vi "test.vi"() -> ()   [LabVIEW 2018]
uses:
  Content/TypeDef/EventTypeDef.ctl
  HASS-LV-WS_integration.lvlib
  <vilib>/MediaMongrels Ltd/WebSockets/WebSockets/WebSockets.lvlib
panel:
  out "States":T1(array[cluster])
  in  "Fetch states":bool
  out "Success":bool
  in  "Call Service Data":T2
  in  "call service btn":bool
  out "Event Data":string
  in  "Remove Button":bool
  in  "Add Button":bool
  in  "Event":string
  out "Event Name":string
  in  "Stop Button":bool
  out "Connection Authenticated?":bool
  out "Connection Result":string
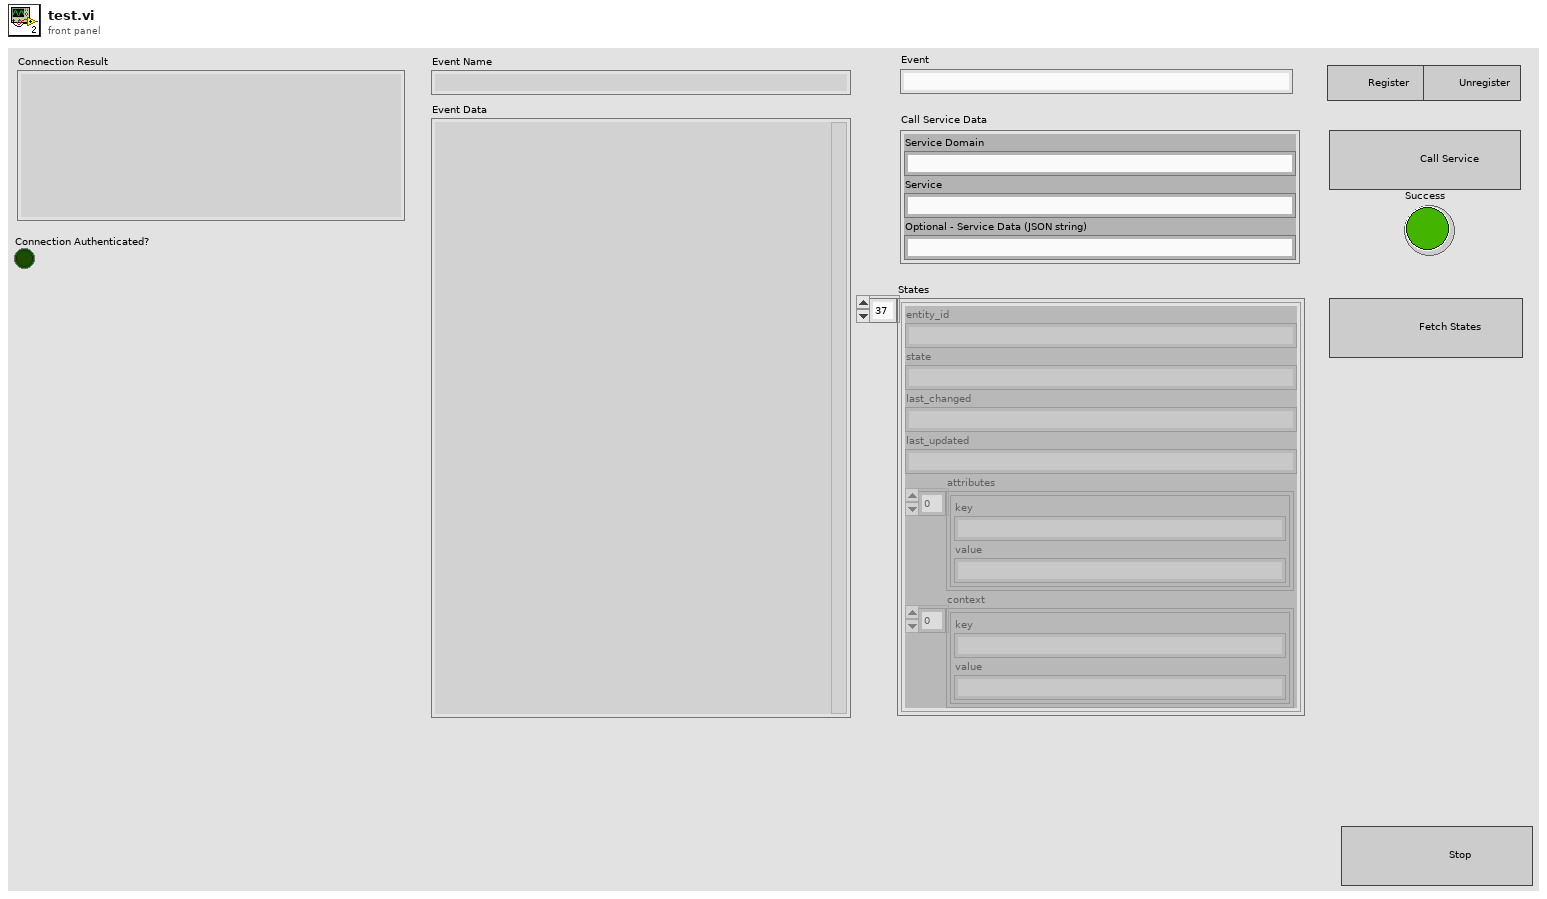
[diagram p1: front panel]
types:
  T1 = cluster{"entity_id":string, "state":string, "last_changed":string, "last_updated":string, "attributes":cluster{"key":string, "value":string}[], "context":cluster{"key":string, "value":string}[]}[]
  T2 = cluster{"Service Domain":string, "Service":string, "Optional - Service Data (JSON string)":string}
  T3 = typedef "HASS-LV-WS_integration.lvlib/ReferencesTypeDef.ctl" = cluster{"user event":refnum<user-event>, "send queue":refnum<queue>, "receive queue":refnum<queue>, "TCP Network Connection":refnum<k5>, "ws engine notifier ":refnum<notifier>, "Event Registration Refnum":refnum<event-registration>}
  T4 = typedef "HASS-LV-WS_integration.lvlib/EventTypeDef.ctl" = cluster{"Data":variant, "Command":string}
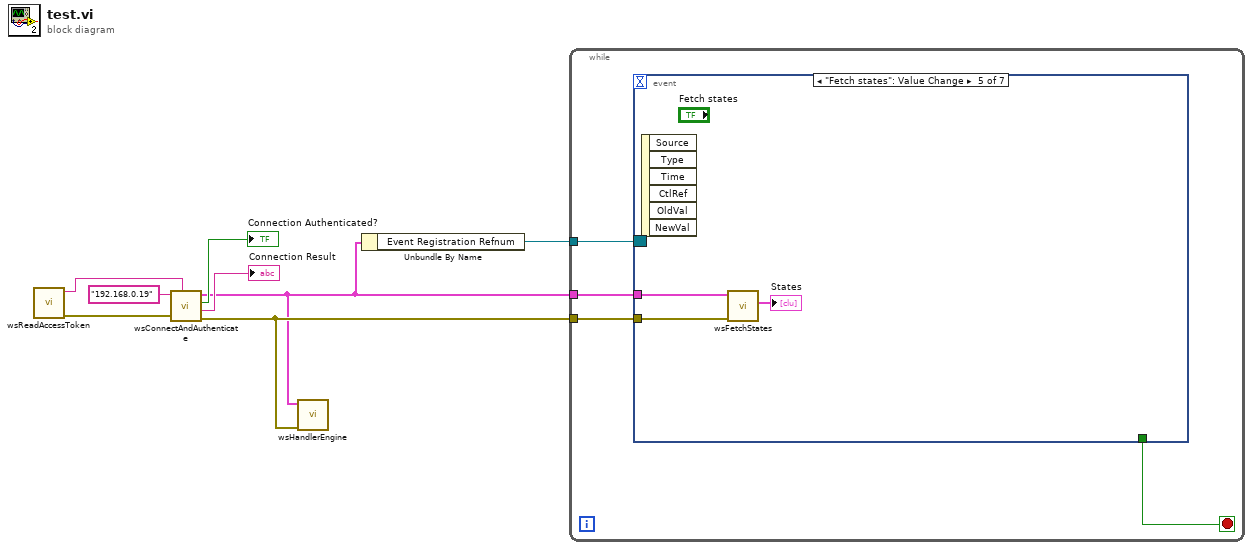
[diagram p0: block diagram]
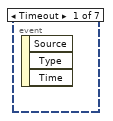
[diagram p2: hidden frame]
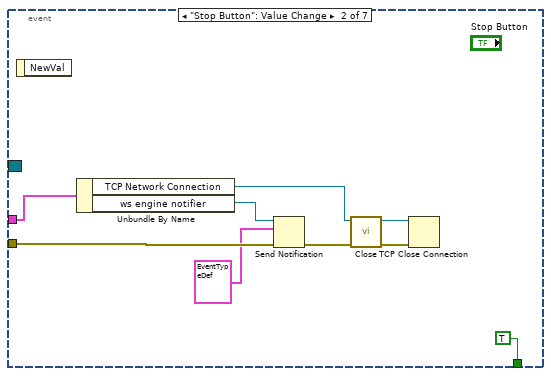
[diagram p3: hidden frame]
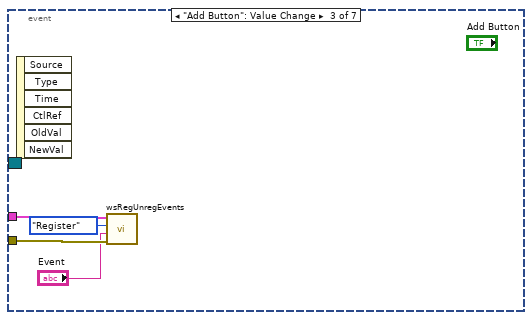
[diagram p4: hidden frame]
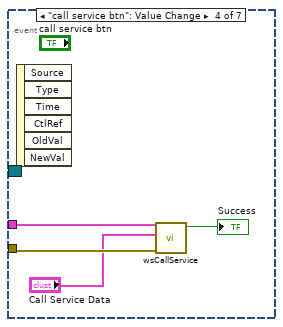
[diagram p5: hidden frame]
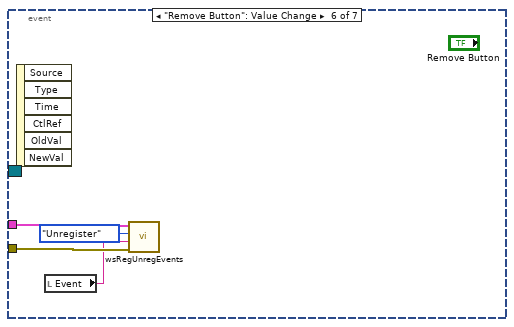
[diagram p6: hidden frame]
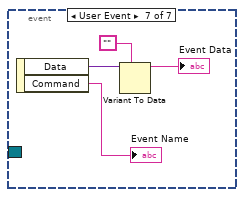
[diagram p7: hidden frame]
diagram:
  n1 = call "wsReadAccessToken.vi"() -> ("error out"=w2:errorcluster, "access token"=w1:string)  [unwired: 9 in, 1 out]
  n2 = call "wsConnectAndAuthenticate.vi"("Access Token"=w1, "error in (no error)"=w2, "Server Address"="192.168.0.19") -> ("error out"=w5:errorcluster, "Connection Result"=→"Connection Result":string, "Connection Authenticated?"=→"Connection Authenticated?":bool, "References"=w3:T3)  [unwired: 5 in]
  n3 = call "wsHandlerEngine.vi"("error in (no error)"=w5, "References"=w3) -> ()  [unwired: 9 in, 1 out]
  n4 = Unbundle By Name(w3) -> ("Event Registration Refnum"=w4:refnum<event-registration>)
  n5 = while {
    tunnel: w3 -> [w11]
    tunnel: w5 -> [w10]
    tunnel: w4 -> [w9]
    stop <- w12 stop-if-true
    n6 = event shown="[4] \"Fetch states\": Value Change" {
      selector: w9 -> [_ _ _ _ _ _ _]
      dyn-events: _ -> [_ _ _ _ _ _ _]
      timeout: _ -> [_ _ _ _ _ _ _]
      tunnel: [_ TRUE _ _ _ _ _] -> w12
      tunnel: w11 -> [_ w20 w25 w28 w31 w35 _]
      tunnel: w10 -> [_ w18 w24 w29 w32 w36 _]
      event Timeout {
        n7 = event-data() -> ()  [unwired: 1 in, 3 out]
      }
      event "Stop Button": Value Change {
        n8 = event-data() -> ()  [unwired: 1 in, 1 out]
        n9 = Unbundle By Name(w20) -> ("TCP Network Connection"=w15:refnum<k5>, "ws engine notifier"=w19:refnum<notifier>)
        n10 = Send Notification(notification=T4 {"Data"=variant, "Command"="Quit"}, notifier=w19, error in (no error)=w18) -> (error out=w17:errorcluster)  [unwired: 1 out]
        n11 = call <vilib>:"Close.vi"("error in (no error)"=w17, "WebSocket Connection in"=w15) -> ("error out"=w16:errorcluster, "WebSocket Connection in"=w14:refnum<k5>)  [unwired: 8 in]
        n12 = TCP Close Connection(connection ID=w14, error in (no error)=w16) -> ()  [unwired: 1 in, 2 out]
      }
      event "Add Button": Value Change {
        n13 = event-data() -> ()  [unwired: 1 in, 6 out]
        n14 = call "wsRegUnregEvents.vi"("Error In"=w24, "Event Name (empty =all)"="Event", "Action"=enum16{"Register", "Unregister"}."Register", "References"=w25) -> ()  [unwired: 7 in, 1 out]
      }
      event "call service btn": Value Change {
        n15 = event-data() -> ()  [unwired: 1 in, 6 out]
        n16 = call "wsCallService.vi"("error in (no error)"=w29, "Call Service Data"="Call Service Data", "References"=w28) -> ("Success?"=→"Success":bool)  [unwired: 7 in, 1 out]
      }
      event "Fetch states": Value Change {
        n17 = event-data() -> ()  [unwired: 1 in, 6 out]
        n18 = call "wsFetchStates.vi"("error in (no error)"=w32, "References"=w31) -> ("states"=→"States":T1)  [unwired: 7 in, 2 out]
      }
      event "Remove Button": Value Change {
        n19 = event-data() -> ()  [unwired: 1 in, 6 out]
        n20 = local read "Event"() -> (w34:string)
        n21 = call "wsRegUnregEvents.vi"("Error In"=w36, "Event Name (empty =all)"=w34, "Action"=enum16{"Register", "Unregister"}."Unregister", "References"=w35) -> ()  [unwired: 7 in, 1 out]
      }
      event User Event {
        n22 = event-data() -> ("Data"=w39:variant, "Command"=→"Event Name":string)  [unwired: 1 in]
        n23 = Variant To Data(type="", Variant=w39) -> (data=→"Event Data":string)  [unwired: 1 in, 1 out]
      }
    }
  }
